vi "BPM.vi"(4 "error in (no error)":errorcluster, 6 "Max BPM Threshold":dbl, 7 "Time Stamp":timestamp) -> (0 "error out":errorcluster, 2 "BPM":dbl, 3 "Below MAX BPM Threshold?":bool)   [LabVIEW 2012]
doc: "Takes the <b>Time Stamp</b> of the last pulse and if the time stamp results in a BPM below <b>Max BPM Threshold</b> then the VI returns the <b>BPM</b> as well as the boolean <b>Below MAX BPM Threshold?</b>"
uses:
  <vilib>/Analysis/baseanly.llb/Mean (DBL).vi
  <vilib>/Analysis/NI_AALBase.lvlib
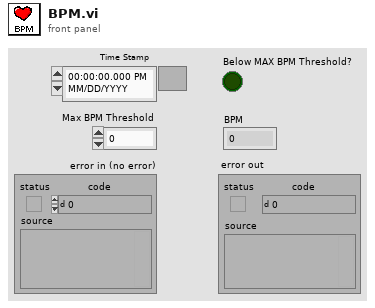
[diagram p1: front panel]
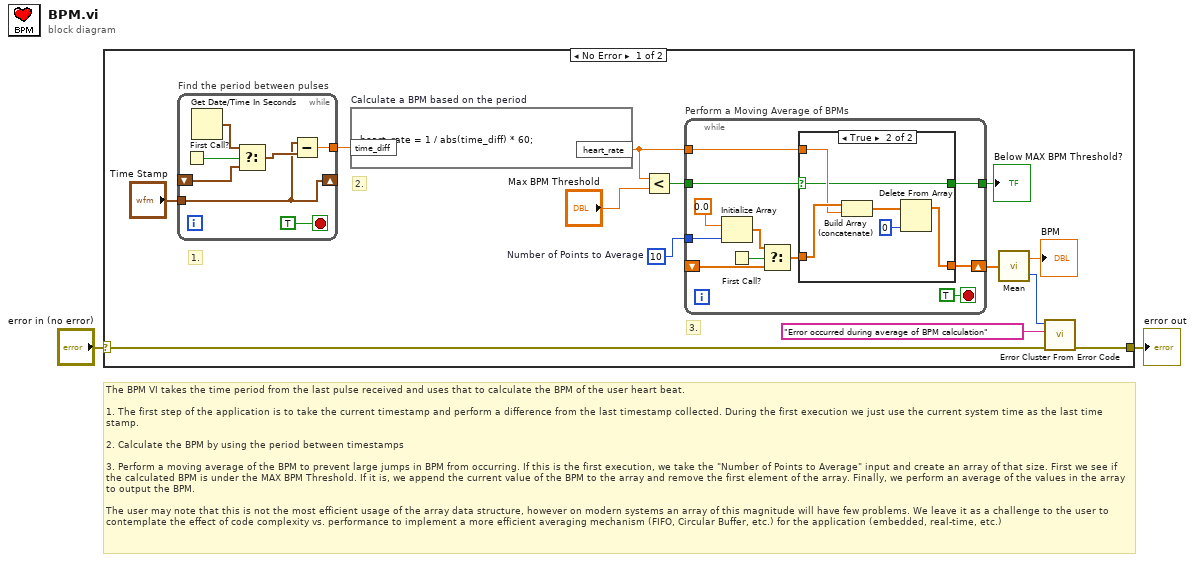
[diagram p0: block diagram]
diagram:
  # "The BPM VI takes the time period from the last pulse received and uses that to calculate the BPM of the user heart beat.\n\n1. The first step of the application is to take the current timestamp and perform a difference from the last timestamp collected. During the first execution we just use the current system time as the last time stamp.\n\n2. Calculate the BPM by using the period between timestamps\n\n3. Perform a moving average of the BPM to prevent large jumps in BPM from occurring. If this is the first execution, we take the \"Number of Points to Average\" input and create an array of that size. First we see if the calculated BPM is under the MAX BPM Threshold. If it is, we append the current value of the BPM to the array and remove the first element of the array. Finally, we perform an average of the values in the array to output the BPM.\n\nThe user may note that this is not the most efficient usage of the array data structure, however on modern systems an array of this magnitude will have few problems. We leave it as a challenge to the user to contemplate the effect of code complexity vs. performance to implement a more efficient averaging mechanism (FIFO, Circular Buffer, etc.) for the application (embedded, real-time, etc.)"
  n1 = case shown="No Error" "error in (no error)" {
    selector: "error in (no error)" -> [w8 w42]
    tunnel: [w9 w42] -> w1
    frame No Error {
      w3 = 10  # Number of Points to Average
      # "3."
      # "2."
      # "1."
      n2 = while "Find the period between pulses" {
        shift-right: [w17] -> _
        shift-left: _ -> [w19]
        tunnel: "Time Stamp" -> [w17]
        tunnel: [w16] -> w14
        stop <- TRUE stop-if-true
        n3 = First Call?() -> (First Call?: T/F=w20:bool)
        n4 = Get Date/Time In Seconds() -> (seconds since 1Jan1904=w21:timestamp)
        n5 = Select(t=w21, s=w20, f=w19) -> (s? t:f=w18:timestamp)
        n6 = Subtract(x=w17, y=w18) -> (x-y=w16:dbl)
      }
      n7 = formula code="heart_rate = 1 / abs(time_diff) * 60;" "Calculate a BPM based on the period"("time_diff"=w14) -> ("heart_rate"=w11:dbl)
      n8 = Less?(x=w11, y="Max BPM Threshold") -> (x < y?=w12:bool)
      n9 = while "Perform a Moving Average of BPMs" {
        tunnel: w12 -> [w27]
        shift-right: [w26] -> w10
        shift-left: _ -> [w31]
        tunnel: w11 -> [w25]
        tunnel: [w24] -> w4
        tunnel: w3 -> [w23]
        stop <- TRUE stop-if-true
        n10 = Initialize Array(0.0 ("element"), w23) -> (w30:dbl[])
        n11 = First Call?() -> (First Call?: T/F=w32:bool)
        n12 = Select(t=w30, s=w32, f=w31) -> (s? t:f=w28:dbl[])
        n13 = case shown="True" w27 {
          selector: w27 -> [w34 w36]
          tunnel: w28 -> [w35 w41]
          tunnel: [w35 w37] -> w26
          tunnel: w25 -> [_ w40]
          tunnel: [w34 w36] -> w24
          frame False {
          }
          frame True {
            n14 = Build Array (concatenate)(w41, w40) -> (w39:dbl[])
            n15 = Delete From Array(array=w39, index=0) -> (array with subset deleted=w37:dbl[])  [unwired: 1 in, 1 out]
          }
        }
      }
      "Below MAX BPM Threshold?" <- w4
      n16 = call-poly <vilib>:"Mean.vi"("X"=w10) -> ("mean"=→"BPM":dbl, "error"=w6:i32)
      n17 = call <vilib>:"Error Cluster From Error Code.vi"("error in (no error)"=w8, "error message (\"\")"="Error occurred during average of BPM calculation" ("error message (\"\")"), "error code (0)"=w6) -> ("error out"=w9:errorcluster)  [unwired: 6 in]
    }
    frame Error {
    }
  }
  "error out" <- w1
